vi "Microchip 93LC56BT Read.vi"() -> ()   [LabVIEW 2015]
doc: "This example shows a more generalized way to use the SPI advanced API to read data. It allows the user to change the following parameters: the endianness of the address bytes, and the number of bytes in an address.\n\nThe parameters will have the following effects:\n\nData Address Width: This will allow the user to specify the EEPROM Data Address as either 1 or 2 bytes.\nData Address Endianness: This control will change the ordering of the bytes in the EEPROM Data Address, note that this only has an effect if there are 2 bytes in the address.\n\nFor connection information see the NI-845x Hardware and Software manual and the manual for your specific SPI device."
uses:
  <vilib>/ni845x/ni845x.llb/ni845xControl.ctl
  <vilib>/ni845x/ni845x.llb/NI-845x SPI Close Script Reference.vi
  <resource>/objmgr/NI845x.rc
panel:
  in  "Target Page Size (bytes)":u32=2
  in  "I/O Voltage Level":i32(ring)=33 items=["3.3V"=33, "2.5V"=25, "1.8V"=18, "1.5V"=15, "1.2V"=12]
  in  "Data Address Width":enum16{"1 Byte", "2 Byte"}(ring)=enum."2 Byte"
  in  "Data Address Endianness":bool=TRUE
  in  "EEPROM Data Address":u8 format="%.0x"
  in  "Number of Bytes to Read":u32=2
  in  "Clock Rate (kHz)":u16=2000
  in  "Chip Select":u32
  out "Read Data":u16[](array[numeric]) format="%x"
  in  "Device":T1="NI-8451"
  # "Device Configuration"
  # "SPI Data"
  # "SPI Slave Configuration"
  # "Note 1: Microchip 93C76/86\nEEPROM devices DC signal levels\nare 2.0V (min) to Vcc (5.0V) +1V\nmax.\n\nNote 2: NI-8451 max signal\nlevel is 3.5V so recommended\nI/O voltage of 3.3V is OK."
  # "Big Endian"
  # "Little Endian"
  # "2048 x 8- or 1024 x 16-bit organization (93C86)"
  # "Clock frequency FCLK — 2 MHz"
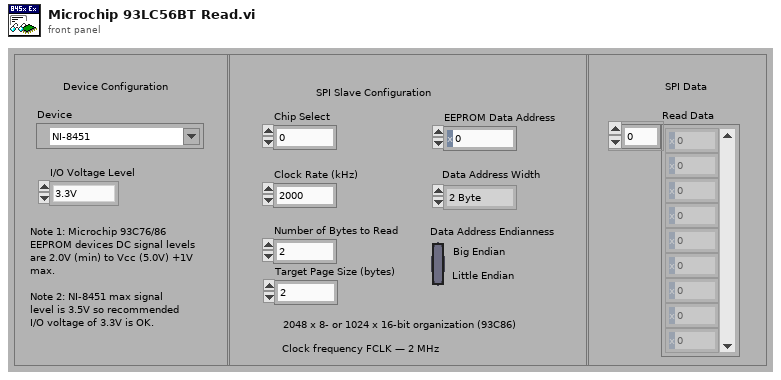
[diagram p1: front panel]
types:
  T1 = typedef "ni845xControl.ctl" = refnum<k21>
  T2 = typedef "ni845xSpiScriptControl.ctl" = refnum<k20>
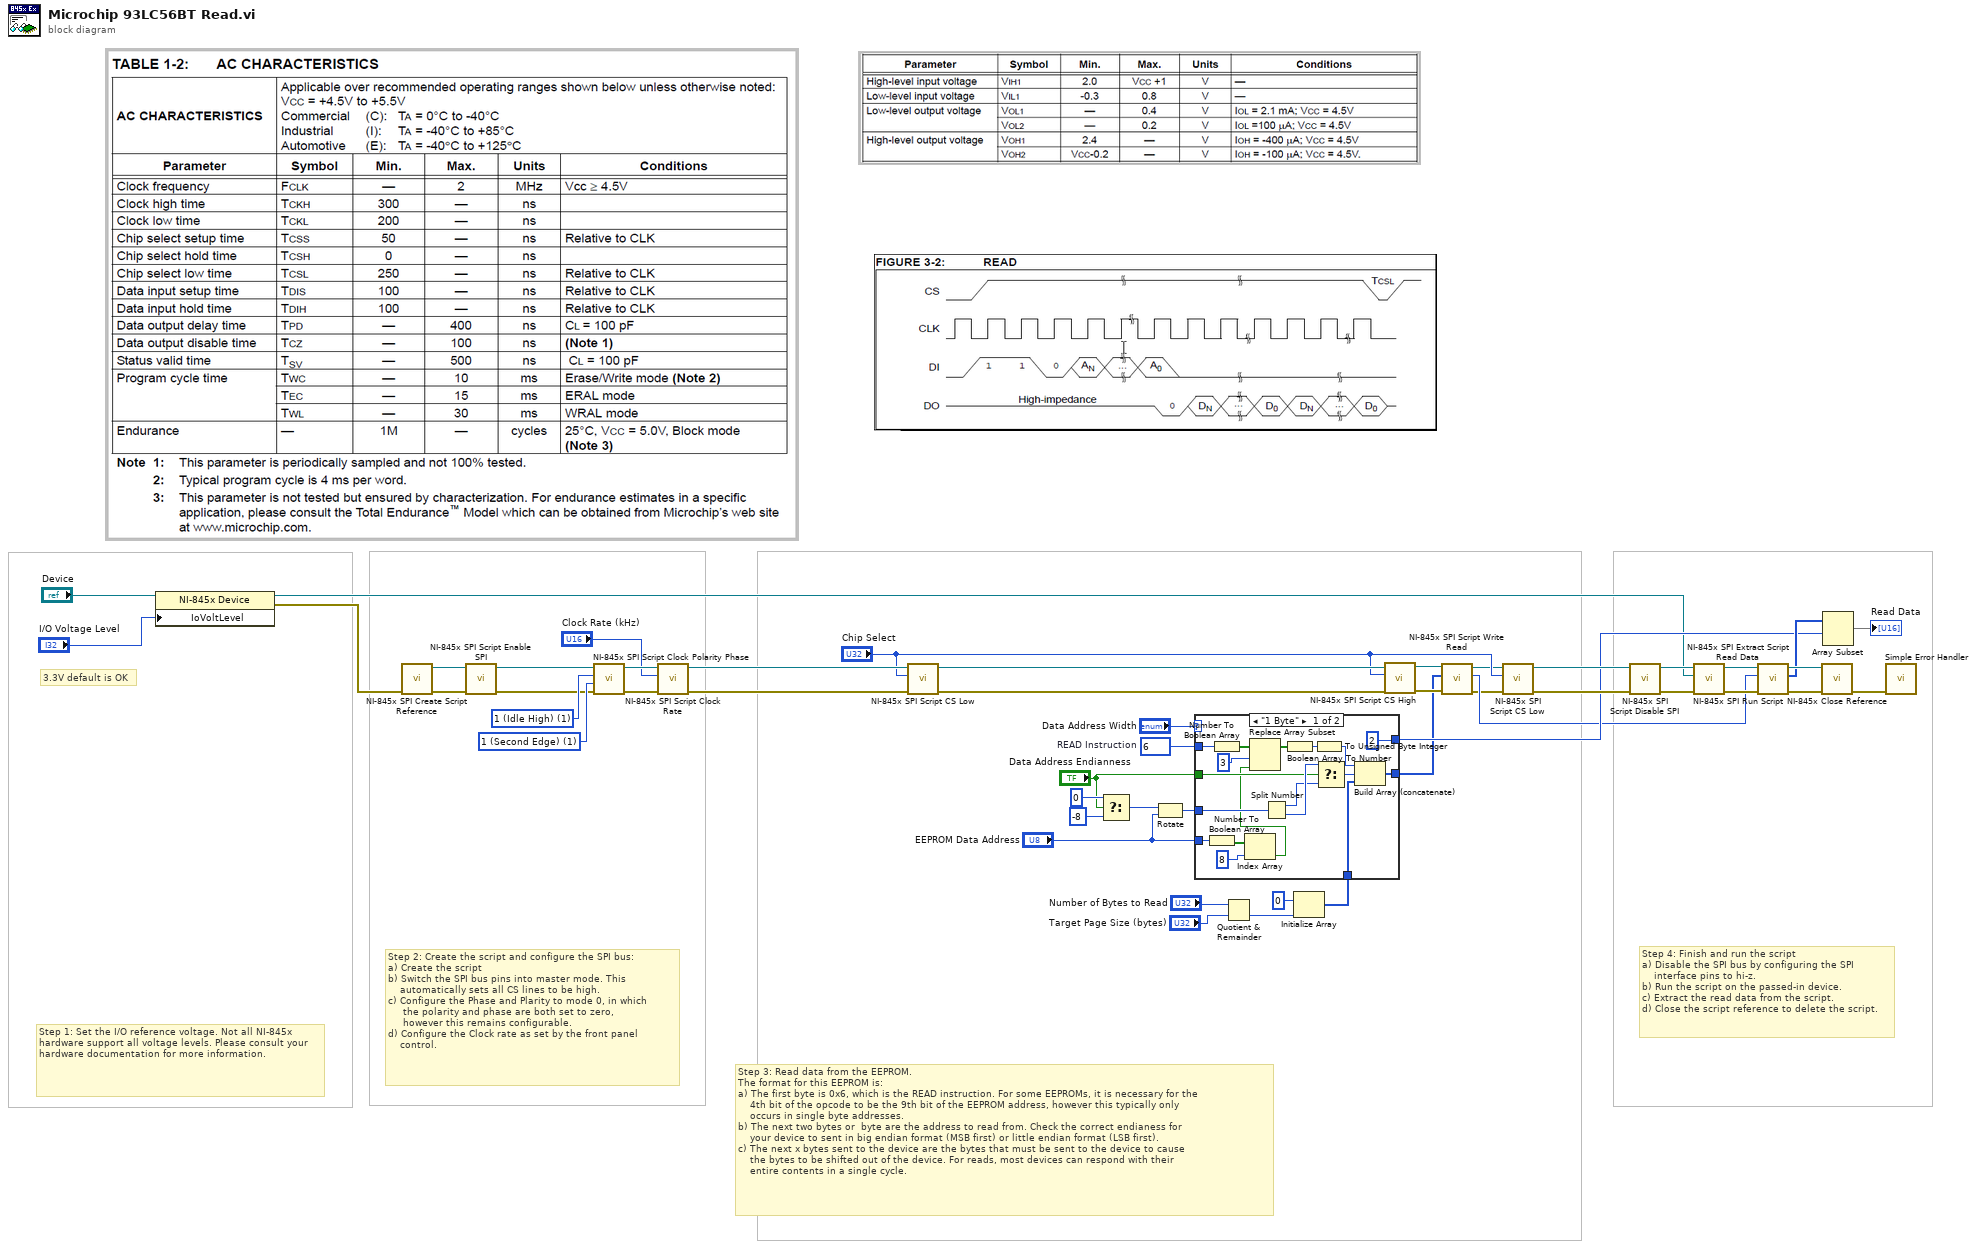
[diagram p0: block diagram]
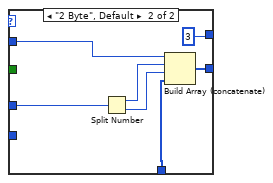
[diagram p2: hidden frame]
diagram:
  w8 = u8 6  # READ Instruction
  w37 = 1 items=["0 (First Edge)", "1 (Second Edge)"] ("clock phase (0)")
  w38 = 1 items=["0 (Idle Low)", "1 (Idle High)"] ("clock polarity (0)")
  # "3.3V default is OK"
  # "Step 1: Set the I/O reference voltage. Not all NI-845x hardware support all voltage levels. Please consult your hardware documentation for more information."
  # "Step 4: Finish and run the script\na) Disable the SPI bus by configuring the SPI \n    interface pins to hi-z.\nb) Run the script on the passed-in device. \nc) Extract the read data from the script.\nd) Close the script reference to delete the script."
  # "Step 3: Read data from the EEPROM. \nThe format for this EEPROM is:\na) The first byte is 0x6, which is the READ instruction. For some EEPROMs, it is necessary for the   \n    4th bit of the opcode to be the 9th bit of the EEPROM address, however this typically only   \n    occurs in single byte addresses.\nb) The next two bytes or  byte are the address to read from. Check the correct endianess for\n    your device to sent in big endian format (MSB first) or little endian format (LSB first).\nc) The next x bytes sent to the device are the bytes that must be sent to the device to cause \n    the bytes to be shifted out of the device. For reads, most devices can respond with their \n    entire contents in a single cycle."
  # "Step 2: Create the script and configure the SPI bus:\na) Create the script\nb) Switch the SPI bus pins into master mode. This\n    automatically sets all CS lines to be high.\nc) Configure the Phase and Plarity to mode 0, in which \n     the polarity and phase are both set to zero,\n     however this remains configurable. \nd) Configure the Clock rate as set by the front panel \n    control."
  n1 = property on="Property Node" class="NI-845x Device"(reference="Device", "IoVoltLevel"="I/O Voltage Level") -> (reference out=w25:T1, error out=w24:errorcluster)  [unwired: 1 in]
  n2 = call <vilib>:"NI-845x SPI Create Script Reference.vi"("error in (no error)"=w24) -> ("error out"=w35:errorcluster, "spi script reference"=w36:T2)  [unwired: 9 out]
  n3 = call <vilib>:"NI-845x SPI Script Enable SPI.vi"("error in (no error)"=w35, "spi script reference in"=w36) -> ("error out"=w33:errorcluster, "spi script reference out"=w34:T2)  [unwired: 8 out]
  n4 = call <vilib>:"NI-845x SPI Script Clock Polarity Phase.vi"("error in (no error)"=w33, "clock phase (0)"=w37, "clock polarity (0)"=w38, "spi script reference in"=w34) -> ("error out"=w47:errorcluster, "spi script reference out"=w46:T2)  [unwired: 2 in, 4 out]
  n5 = call <vilib>:"NI-845x SPI Script Clock Rate.vi"("error in (no error)"=w47, "clock rate in kHz (1000)"="Clock Rate (kHz)", "spi script reference in"=w46) -> ("error out"=w42:errorcluster, "spi script reference out"=w41:T2)  [unwired: 1 in, 6 out]
  n6 = call <vilib>:"NI-845x SPI Script CS Low.vi"("error in (no error)"=w42, "chip select (0)"="Chip Select", "spi script reference in"=w41) -> ("error out"=w22:errorcluster, "spi script reference out"=w21:T2)  [unwired: 1 in, 6 out]
  n7 = Select(t=i16 0, s="Data Address Endianness", f=i16 -8) -> (s? t:f=w11:i16)
  n8 = Rotate(1:"EEPROM Data Address", 2:w11) -> (0:w9:u8)
  n9 = Quotient & Remainder(x="Number of Bytes to Read", y="Target Page Size (bytes)") -> (floor(x/y)=w2:u32)  [unwired: 1 out]
  n10 = Initialize Array(u32 0 ("element"), w2) -> (w6:u32[])
  n11 = case shown="\"1 Byte\"" "Data Address Width" {
    tunnel: w9 -> [w66 w72]
    tunnel: [w67 w70] -> w14
    tunnel: w8 -> [w61 w71]
    tunnel: "Data Address Endianness" -> [w62 _]
    tunnel: w6 -> [w50 w68]
    tunnel: [2 ("index") 3 ("index")] -> w27
    tunnel: "EEPROM Data Address" -> [w52 _]
    frame "1 Byte" {
      n12 = Number To Boolean Array(number=w52) -> (Boolean array=w54:bool[])
      n13 = Number To Boolean Array(number=w61) -> (Boolean array=w60:bool[])
      n14 = Index Array(array=w54, index=8) -> (element=w53:bool)
      n15 = Replace Array Subset(array=w60, new element=w53, index=3) -> (w58:bool[])
      n16 = Split Number(x=w66) -> (hi(x)=w64:u8, lo(x)=w65:u8)
      n17 = Boolean Array To Number(Boolean array=w58) -> (number=w57:u32)
      n18 = To Unsigned Byte Integer(number=w57) -> (unsigned 8bit integer=w56:u8)
      n19 = Select(t=w65, s=w62, f=w64) -> (s? t:f=w63:u8)
      n20 = Build Array (concatenate)(w56, w63, w50) -> (w67:u32[])
    }
    frame "2 Byte", Default {
      n21 = Split Number(x=w72) -> (hi(x)=w74:u8, lo(x)=w73:u8)
      n22 = Build Array (concatenate)(w71, w74, w73, w68) -> (w70:u32[])
    }
  }
  n23 = call <vilib>:"NI-845x SPI Script CS High.vi"("error in (no error)"=w22, "chip select (0)"="Chip Select", "spi script reference in"=w21) -> ("error out"=w16:errorcluster, "spi script reference out"=w15:T2)  [unwired: 7 in]
  n24 = call <vilib>:"NI-845x SPI Script Write Read.vi"("error in (no error)"=w16, "write data"=w14, "spi script reference in"=w15) -> ("error out"=w18:errorcluster, "script read index"=w19:u32, "spi script reference out"=w17:T2)  [unwired: 1 in, 5 out]
  n25 = call <vilib>:"NI-845x SPI Script CS Low.vi"("error in (no error)"=w18, "chip select (0)"="Chip Select", "spi script reference in"=w17) -> ("error out"=w48:errorcluster, "spi script reference out"=w45:T2)  [unwired: 7 in]
  n26 = call <vilib>:"NI-845x SPI Script Disable SPI.vi"("error in (no error)"=w48, "spi script reference in"=w45) -> ("error out"=w49:errorcluster, "spi script reference out"=w44:T2)  [unwired: 8 out]
  n27 = call <vilib>:"NI-845x SPI Run Script.vi"("error in (no error)"=w49, "device reference in"=w25, "spi script reference in"=w44) -> ("error out"=w40:errorcluster, "spi script reference out"=w39:T2)  [unwired: 1 in, 6 out]
  n28 = call <vilib>:"NI-845x SPI Extract Script Read Data.vi"("error in (no error)"=w40, "script read index"=w19, "spi script reference in"=w39) -> ("error out"=w31:errorcluster, "read data"=w28:u8[], "spi script reference out"=w32:T2)  [unwired: 6 out]
  n29 = call-poly <vilib>:"NI-845x Close Reference.vi"("error in (no error)"=w31, "spi script reference"=w32) -> ("error out"=w30:errorcluster)  [unwired: 9 out]
  n30 = Array Subset(array=w28, index=w27) -> (→"Read Data":u8[])  [unwired: 1 in]
  n31 = call <vilib>:"Simple Error Handler.vi"("error in (no error)"=w30) -> ()  [unwired: 1 in, 8 out]
